vi "Generate Signature.vi"(8 "error in (no error)":errorcluster, 9 "Key":string, 10 "Message":string, 11 "Signature in":refnum<class "Signature.lvclass">) -> (0 "error out":errorcluster, 2 "Signature":string, 3 "Signature out":refnum<class "Signature.lvclass">)   [LabVIEW 2017, in "Crypto.lvlib" / "Signature.lvclass"]
uses:
  Signature.lvclass
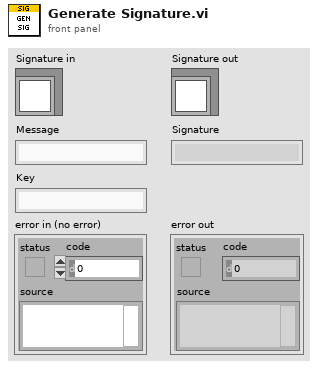
[diagram p1: front panel]
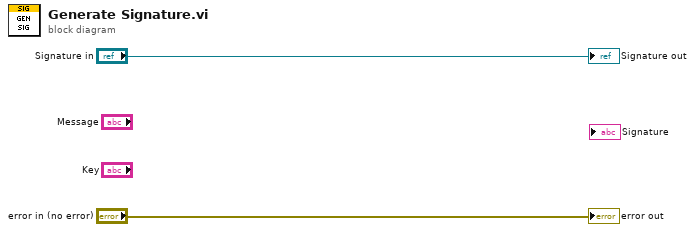
[diagram p0: block diagram]
diagram:
  "error out" <- "error in (no error)"
  "Signature out" <- "Signature in"
